vi "Current ranging routine (SubVI).vi"(11 "Current":dbl) -> ()   [LabVIEW 2020]
uses:
  Labview/IVIUM/IVIUM_remdriver.lvlib
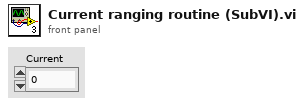
[diagram p1: front panel]
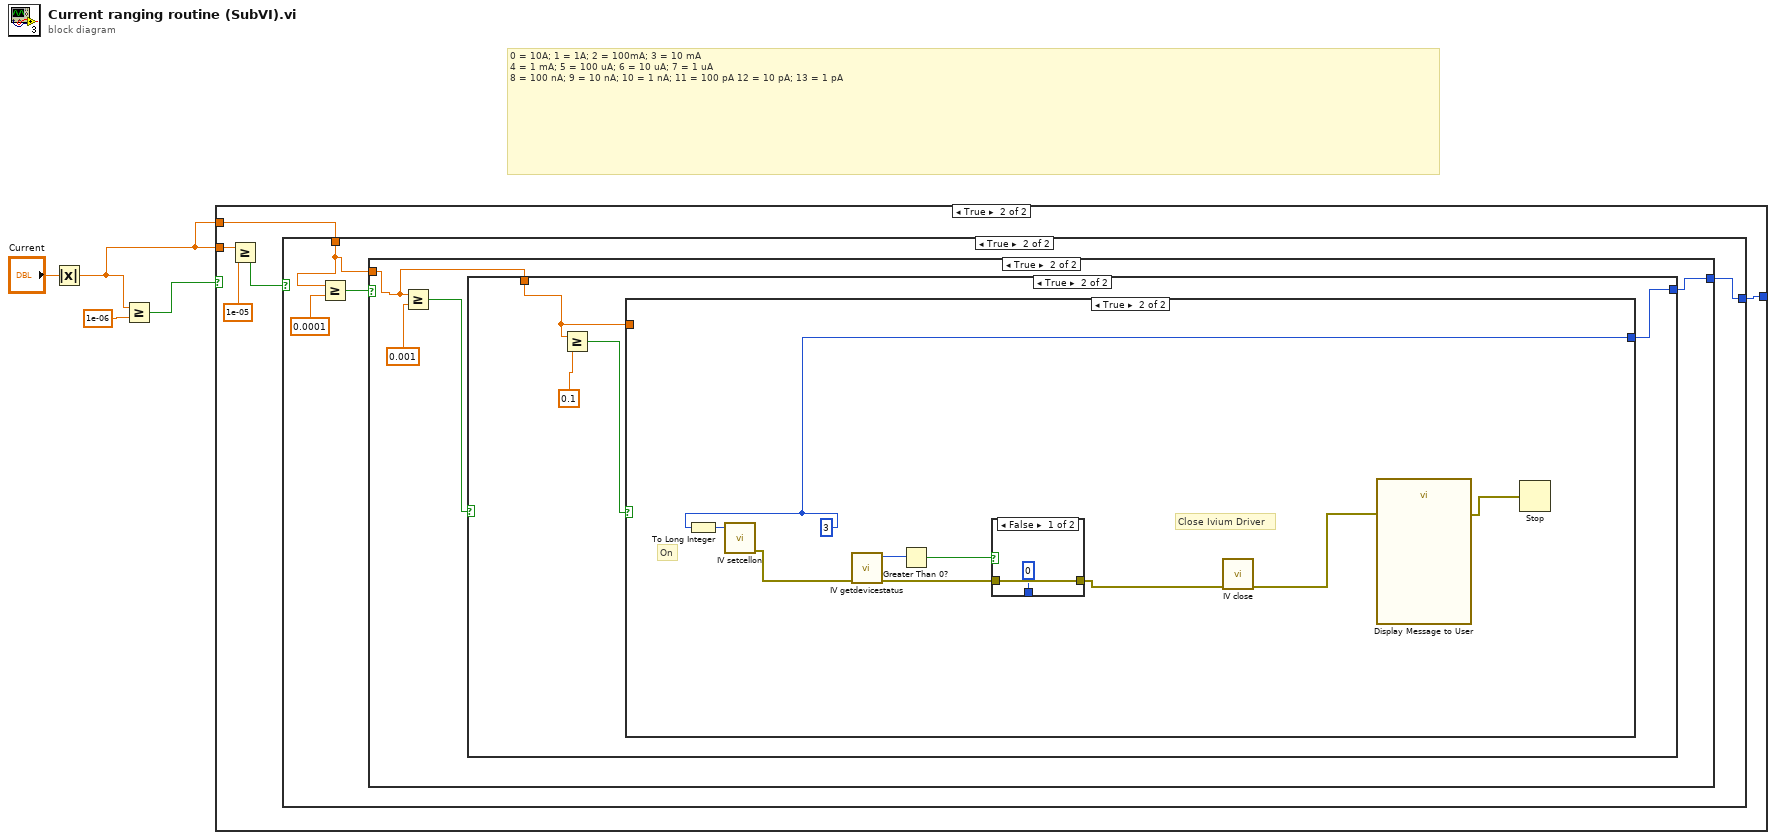
[diagram p0: block diagram]
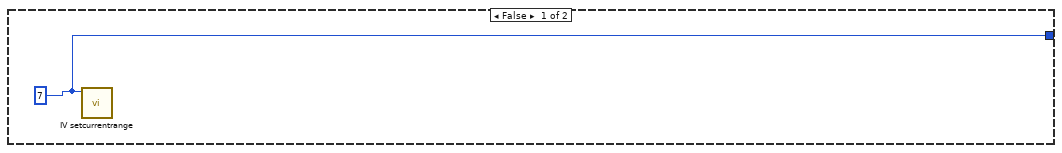
[diagram p2: hidden frame]
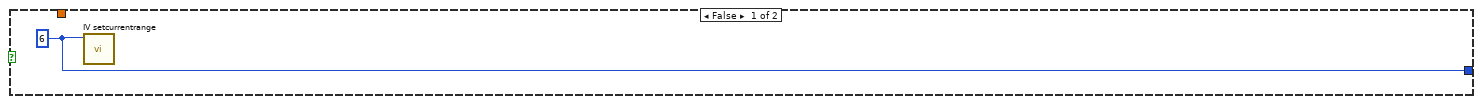
[diagram p3: hidden frame]
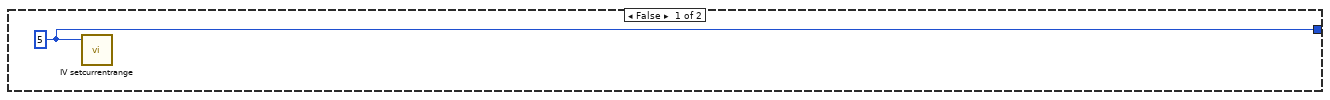
[diagram p4: hidden frame]
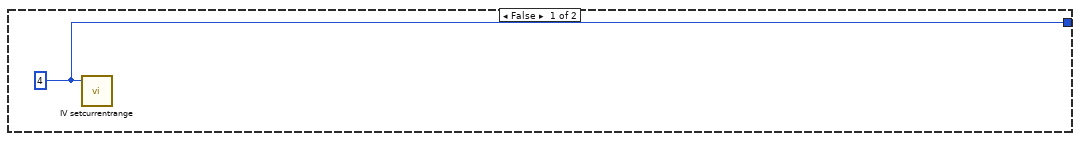
[diagram p5: hidden frame]
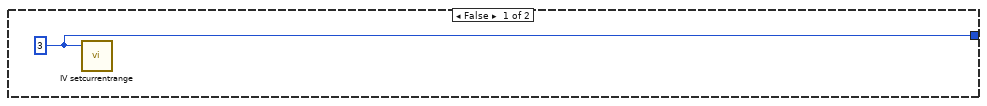
[diagram p6: hidden frame]
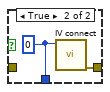
[diagram p7: hidden frame]
diagram:
  # "0 = 10A; 1 = 1A; 2 = 100mA; 3 = 10 mA\n4 = 1 mA; 5 = 100 uA; 6 = 10 uA; 7 = 1 uA\n8 = 100 nA; 9 = 10 nA; 10 = 1 nA; 11 = 100 pA 12 = 10 pA; 13 = 1 pA"
  n1 = Absolute Value(x="Current") -> (abs(x)=w1:dbl)
  n2 = Greater Or Equal?(x=w1, y=1e-06) -> (x >= y?=w4:bool)
  n3 = case shown="True" w4 {
    tunnel: w1 -> [_ w8]
    tunnel: w1 -> [_ w7]
    tunnel: [w5 w6] -> _
    frame False {
      w5 = 7 ("value")
      n4 = call "IV setcurrentrange.vi"("value"=w5) -> ()  [unwired: 8 in, 3 out]
    }
    frame True {
      n5 = Greater Or Equal?(x=w8, y=1e-05 ("x")) -> (x >= y?=w10:bool)
      n6 = case shown="True" w10 {
        tunnel: w7 -> [_ w14]
        tunnel: [w11 w12] -> w6
        frame False {
          w11 = 6 ("value")
          n7 = call "IV setcurrentrange.vi"("value"=w11) -> ()  [unwired: 8 in, 3 out]
        }
        frame True {
          n8 = Greater Or Equal?(x=w14, y=0.0001 ("x")) -> (x >= y?=w13:bool)
          n9 = case shown="True" w13 {
            tunnel: w14 -> [_ w18]
            tunnel: [w16 w17] -> w12
            frame False {
              w16 = 5 ("value")
              n10 = call "IV setcurrentrange.vi"("value"=w16) -> ()  [unwired: 8 in, 3 out]
            }
            frame True {
              n11 = Greater Or Equal?(x=w18, y=0.001 ("x")) -> (x >= y?=w19:bool)
              n12 = case shown="True" w19 {
                tunnel: w18 -> [_ w23]
                tunnel: [w21 w22] -> w17
                frame False {
                  w21 = 4 ("value")
                  n13 = call "IV setcurrentrange.vi"("value"=w21) -> ()  [unwired: 8 in, 3 out]
                }
                frame True {
                  n14 = Greater Or Equal?(x=w23, y=0.1 ("x")) -> (x >= y?=w24:bool)
                  n15 = case shown="True" w24 {
                    tunnel: w23 -> [_ _]
                    tunnel: [w26 w27] -> w22
                    frame False {
                      w26 = 3 ("value")
                      n16 = call "IV setcurrentrange.vi"("value"=w26) -> ()  [unwired: 8 in, 3 out]
                    }
                    frame True {
                      w27 = 3 ("number")
                      # "Close Ivium Driver"
                      # "On"
                      n17 = To Long Integer(number=w27) -> (32bit integer=w35:i32)
                      n18 = call "IV setcellon.vi"("cellon"=w35) -> ("error out"=w31:errorcluster)  [unwired: 8 in, 2 out]
                      n19 = call "IV getdevicestatus.vi"("error in (no error)"=w31) -> ("error out"=w32:errorcluster, "return type"=w34:i32)  [unwired: 9 in]
                      n20 = Greater Than 0?(x=w34) -> (x > 0?=w33:bool)
                      n21 = case shown="False" w33 {
                        tunnel: [w37 w39] -> w30
                        tunnel: w32 -> [w37 _]
                        tunnel: [0 ("devconnect") w38] -> _
                        frame False {
                        }
                        frame True {
                          w38 = 0 ("devconnect")
                          n22 = call "IV connect.vi"("devconnect"=w38) -> ("error out"=w39:errorcluster)  [unwired: 8 in, 2 out]
                        }
                      }
                      n23 = call "IV close.vi"("error in (no error)"=w30) -> ("error out"=w29:errorcluster)  [unwired: 9 in, 1 out]
                      n24 = call "Display Message to User"("error in (no error)"=w29) -> ("error out"=w28:errorcluster)  [unwired: 9 in, 1 out]
                      n25 = Stop(stop? (T)=w28) -> ()
                    }
                  }
                }
              }
            }
          }
        }
      }
    }
  }
